vi "read.vi"(8 "error in (no error)":errorcluster, 11 "SerialReal in":refnum<class "SerialReal.lvclass">) -> (0 "error out":errorcluster, 2 "stringRead":string, 3 "SerialReal out":refnum<class "SerialReal.lvclass">)   [LabVIEW 2012, in "SerialProtocols.lvlib" / "SerialReal.lvclass"]
uses:
  SerialReal.lvclass
  SerialReal.lvclass/SerialReal.ctl
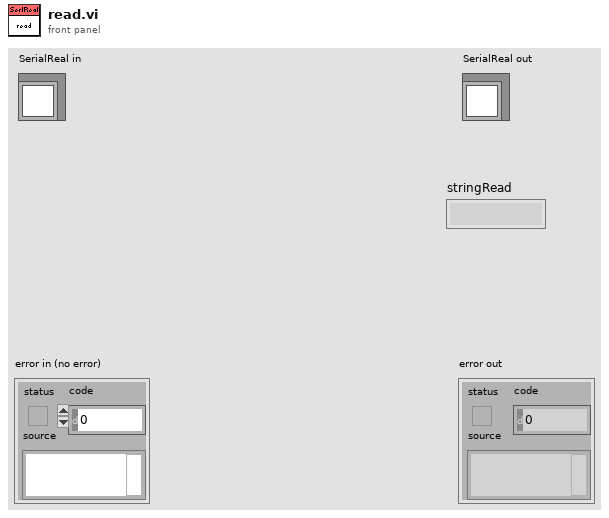
[diagram p1: front panel]
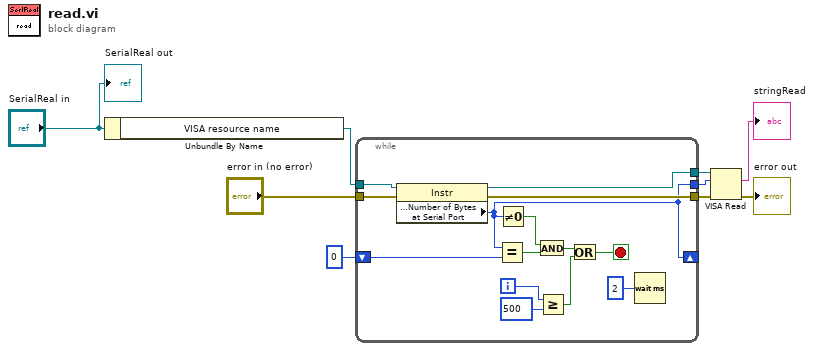
[diagram p0: block diagram]
diagram:
  n1 = Unbundle By Name("SerialReal in") -> ("VISA resource name"=w8:refnum<visa-resource-name>)
  n2 = while {
    tunnel: w8 -> [w23]
    tunnel: "error in (no error)" -> [w22]
    tunnel: [w21] -> w6
    tunnel: [w20] -> w5
    tunnel: [w10] -> w4
    shift-right: [w10] -> _
    shift-left: u32 0 ("Bytes at Port") -> [w17]
    i -> [w13]
    stop <- w11 stop-if-true
    n3 = property class="Instr"(reference=w23, error in=w22) -> (reference out=w20:refnum<visa-resource-name>, error out=w21:errorcluster, "Serial Settings:Number of Bytes at Serial Port"=w10:u32)
    n4 = Equal?(x=w10, y=w17) -> (x = y?=w16:bool)
    n5 = Not Equal To 0?(x=w10) -> (x != 0?=w18:bool)
    n6 = And(x=w18, y=w16) -> (x .and. y?=w15:bool)
    n7 = Greater Or Equal?(x=w13, y=500) -> (x >= y?=w14:bool)
    n8 = Or(x=w15, y=w14) -> (x .or. y?=w11:bool)
    n9 = Wait (ms)(milliseconds to wait=u32 2) -> ()  [unwired: 1 out]
  }
  n10 = VISA Read(VISA resource name=w5, byte count=w4, error in (no error)=w6) -> (read buffer=→"stringRead":string, error out=→"error out":errorcluster)  [unwired: 2 out]
  "SerialReal out" <- "SerialReal in"
